vi "Tabbed FP.vi"() -> ()   [LabVIEW 2019]
panel:
  in  "Tab Control":enum32{"Page 1", "Page 2", "Page 3"}(tab)
  out "Boolean":bool
  in  "String":string
  in  "Numeric":dbl
  out "Meter":dbl(knob) scale=0.0..10.0
  in  "Tab Control 2":enum32{"Page 1", "Page 2"}(tab)
  in  "Tab Control 5":enum32{"Page 1", "Page 2"}(tab)
  in  "Tab Control 4":enum32{"Page 1", "Page 2"}(tab)
  in  "Tab Control 3":enum32{"Page 1", "Page 2"}(tab)
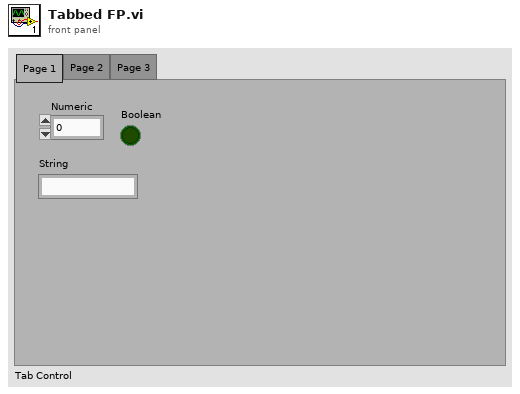
[diagram p1: front panel]
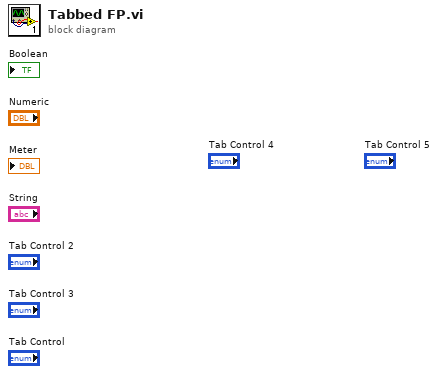
[diagram p0: block diagram]
diagram:
